vi "Prep_Motors_Global_test.vi"(0 "B-Axis":refnum<k7>, 1 "Y-Axis":refnum<k7>, 3 "Z-Axis":refnum<k7>, 4 "X-Axis":refnum<k7>, 5 "Error In":errorcluster) -> (2 "Error Out":errorcluster)   [LabVIEW 2016]
uses:
  Utility/Global_Stage.vi
panel:
  in  "S/N B-Axis":i32=94865857
  in  "S/N Y-Axis":i32=83860202
  in  "S/N X-Axis":i32=83855365
  in  "S/N Z-Axis":i32=83860012
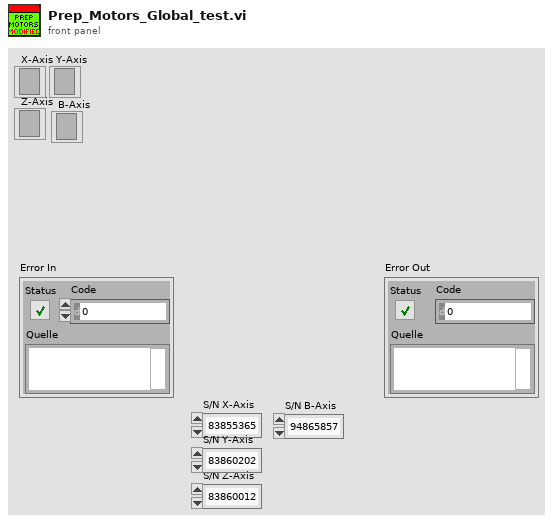
[diagram p1: front panel]
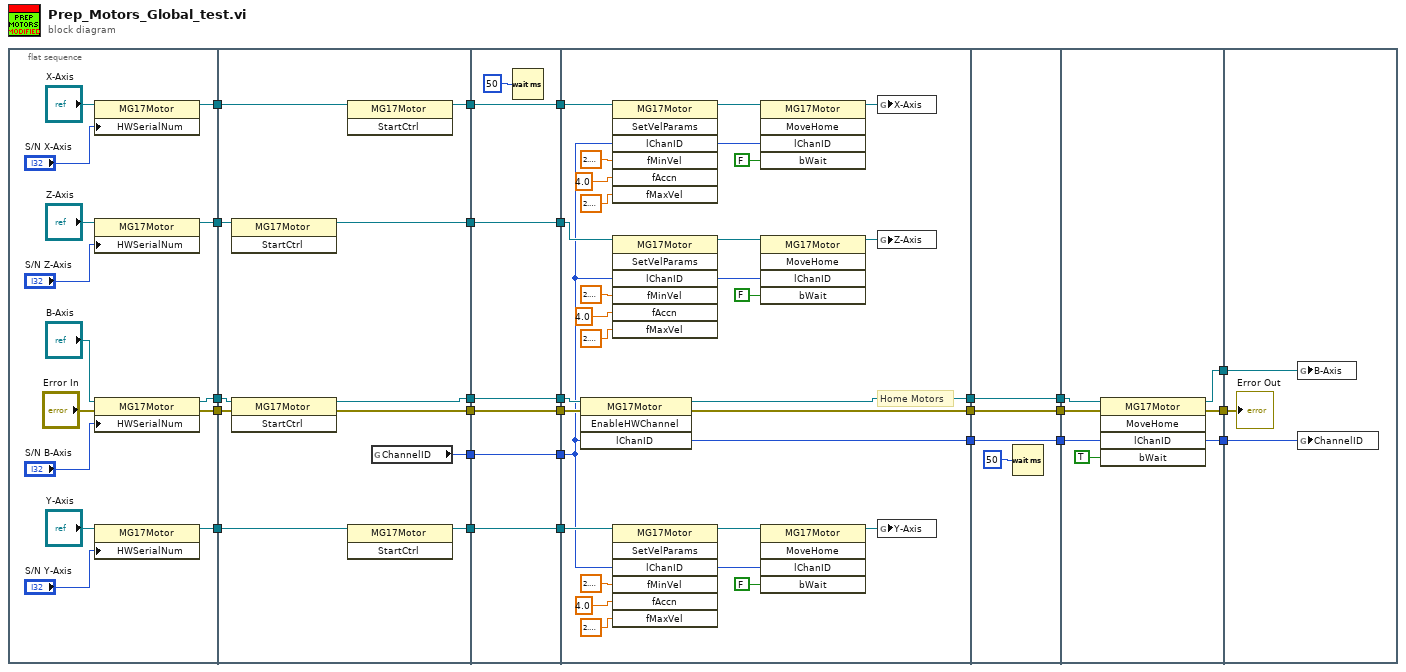
[diagram p0: block diagram]
diagram:
  n1 = flat-sequence {
    tunnel: [w40] -> w26
    tunnel: [w39] -> w25
    tunnel: [w38] -> w24
    tunnel: [w29] -> w23
    tunnel: [w27] -> w22
    tunnel: [w51] -> w21
    tunnel: [w50] -> w19
    tunnel: [w49] -> w17
    tunnel: w26 -> [w48]
    tunnel: w25 -> [w47]
    tunnel: w24 -> [w46]
    tunnel: w23 -> [w45]
    tunnel: [w43] -> w15
    tunnel: w22 -> [w44]
    tunnel: [w42] -> w13
    tunnel: [w41] -> w11
    tunnel: w21 -> [w58]
    tunnel: [w58] -> w20
    tunnel: w19 -> [w57]
    tunnel: [w57] -> w18
    tunnel: w17 -> [w56]
    tunnel: [w56] -> w16
    tunnel: w15 -> [w55]
    tunnel: [w55] -> w14
    tunnel: w13 -> [w54]
    tunnel: [w54] -> w12
    tunnel: w11 -> [w53]
    tunnel: [w53] -> w10
    tunnel: w20 -> [w68]
    tunnel: w18 -> [w66]
    tunnel: w16 -> [w82]
    tunnel: w14 -> [w64]
    tunnel: [w61] -> w9
    tunnel: [w63] -> w8
    tunnel: [w59] -> w7
    tunnel: w12 -> [w62]
    tunnel: w10 -> [w60]
    tunnel: w9 -> [w90]
    tunnel: [w90] -> w6
    tunnel: w8 -> [w89]
    tunnel: [w89] -> w4
    tunnel: w7 -> [w91]
    tunnel: [w91] -> w2
    tunnel: w6 -> [w97]
    tunnel: [w94] -> w5
    tunnel: w4 -> [w96]
    tunnel: [w95] -> w3
    tunnel: w2 -> [w98]
    tunnel: [w93] -> w1
    tunnel: w5 -> [w101]
    tunnel: w3 -> [w100]
    tunnel: w1 -> [w102]
    frame #0 {
      n2 = property on="Eigenschaftsknoten" class="MG17Motor"(reference="X-Axis", "HWSerialNum"="S/N X-Axis") -> (reference out=w40:refnum<k7>)  [unwired: 1 in, 1 out]
      n3 = property on="Eigenschaftsknoten" class="MG17Motor"(reference="Z-Axis", "HWSerialNum"="S/N Z-Axis") -> (reference out=w38:refnum<k7>)  [unwired: 1 in, 1 out]
      n4 = property on="Eigenschaftsknoten" class="MG17Motor"(reference="B-Axis", error in="Error In", "HWSerialNum"="S/N B-Axis") -> (reference out=w29:refnum<k7>, error out=w27:errorcluster)
      n5 = property on="Eigenschaftsknoten" class="MG17Motor"(reference="Y-Axis", "HWSerialNum"="S/N Y-Axis") -> (reference out=w39:refnum<k7>)  [unwired: 1 in, 1 out]
    }
    frame #1 {
      n6 = invoke class="MG17Motor" method="StartCtrl"(reference=w46) -> (reference out=w49:refnum<k7>)  [unwired: 2 in, 2 out]
      n7 = invoke class="MG17Motor" method="StartCtrl"(reference=w45, error in=w44) -> (reference out=w43:refnum<k7>, error out=w42:errorcluster)  [unwired: 1 in, 1 out]
      n8 = invoke class="MG17Motor" method="StartCtrl"(reference=w48) -> (reference out=w51:refnum<k7>)  [unwired: 2 in, 2 out]
      n9 = invoke class="MG17Motor" method="StartCtrl"(reference=w47) -> (reference out=w50:refnum<k7>)  [unwired: 2 in, 2 out]
      n10 = global read "Global_Stage.vi" "ChannelID"() -> (w41:i32)
    }
    frame #2 {
      n11 = Wait (ms)(milliseconds to wait=u32 50) -> ()  [unwired: 1 out]
    }
    frame #3 {
      # "Home Motors"
      n12 = invoke class="MG17Motor" method="EnableHWChannel"(reference=w64, error in=w62, "lChanID"=w60) -> (reference out=w63:refnum<k7>, error out=w61:errorcluster, "lChanID"=w59:i32)  [unwired: 1 in, 1 out]
      n13 = invoke class="MG17Motor" method="SetVelParams"(reference=w68, "lChanID"=w60, "fMinVel"=sgl 2.3, "fAccn"=sgl 4.0, "fMaxVel"=sgl 2.3) -> (reference out=w67:refnum<k7>, "lChanID"=w70:i32)  [unwired: 2 in, 5 out]
      n14 = invoke class="MG17Motor" method="SetVelParams"(reference=w82, "lChanID"=w60, "fMinVel"=sgl 2.3, "fAccn"=sgl 4.0, "fMaxVel"=sgl 2.3) -> (reference out=w81:refnum<k7>, "lChanID"=w77:i32)  [unwired: 2 in, 5 out]
      n15 = invoke class="MG17Motor" method="SetVelParams"(reference=w66, "lChanID"=w60, "fMinVel"=sgl 2.3, "fAccn"=sgl 4.0, "fMaxVel"=sgl 2.3) -> (reference out=w65:refnum<k7>, "lChanID"=w69:i32)  [unwired: 2 in, 5 out]
      n16 = invoke class="MG17Motor" method="MoveHome"(reference=w67, "lChanID"=w70, "bWait"=FALSE) -> (reference out=w84:refnum<k7>)  [unwired: 2 in, 4 out]
      n17 = invoke class="MG17Motor" method="MoveHome"(reference=w81, "lChanID"=w77, "bWait"=FALSE) -> (reference out=w85:refnum<k7>)  [unwired: 2 in, 4 out]
      n18 = invoke class="MG17Motor" method="MoveHome"(reference=w65, "lChanID"=w69, "bWait"=FALSE) -> (reference out=w83:refnum<k7>)  [unwired: 2 in, 4 out]
      n19 = global write "Global_Stage.vi" "X-Axis"(w84) -> ()
      n20 = global write "Global_Stage.vi" "Z-Axis"(w85) -> ()
      n21 = global write "Global_Stage.vi" "Y-Axis"(w83) -> ()
    }
    frame #4 {
      n22 = Wait (ms)(milliseconds to wait=u32 50) -> ()  [unwired: 1 out]
    }
    frame #5 {
      n23 = invoke class="MG17Motor" method="MoveHome"(reference=w96, error in=w97, "lChanID"=w98, "bWait"=TRUE) -> (reference out=w95:refnum<k7>, error out=w94:errorcluster, "lChanID"=w93:i32)  [unwired: 1 in, 2 out]
    }
    frame #6 {
      n24 = global write "Global_Stage.vi" "B-Axis"(w100) -> ()
      n25 = global write "Global_Stage.vi" "ChannelID"(w102) -> ()
      "Error Out" <- w101
    }
  }
